vi "Next Buffer Size.vi"(3 "Min Size":i32=5, 4 "Times":u32[](array[numeric]), 5 "Buffer Duration (s)":dbl=2.0) -> (0 "Frequency (Hz)":dbl, 2 "Next buffer size":i32)   [LabVIEW 2009]
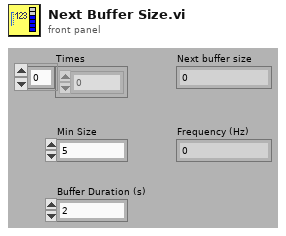
[diagram p1: front panel]
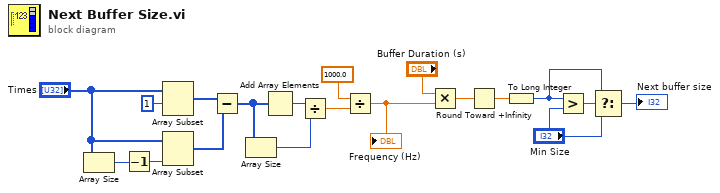
[diagram p0: block diagram]
diagram:
  n1 = Array Size(array="Times") -> (size(s)=w6:i32)
  n2 = Decrement(x=w6) -> (x-1=w5:i32)
  n3 = Array Subset(array="Times", index=1) -> (w10:u32[])  [unwired: 1 in]
  n4 = Array Subset(array="Times", length=w5) -> (w11:u32[])  [unwired: 1 in]
  n5 = Subtract(x=w10, y=w11) -> (x-y=w12:u32[])
  n6 = Array Size(array=w12) -> (size(s)=w14:i32)
  n7 = Add Array Elements(numeric array=w12) -> (sum=w13:u32)
  n8 = Divide(x=w13, y=w14) -> (x/y=w15:dbl)
  n9 = Divide(x=1000.0, y=w15) -> (x/y=w2:dbl)
  "Frequency (Hz)" <- w2
  n10 = Multiply(x="Buffer Duration (s)", y=w2) -> (x*y=w1:dbl)
  n11 = Round Toward +Infinity(x=w1) -> (ceil(x): smallest int >= x=w8:dbl)
  n12 = To Long Integer(number=w8) -> (32bit integer=w7:i32)
  n13 = Greater?(x=w7, y="Min Size") -> (0:w17:bool)
  n14 = Select(t=w7, s=w17, f="Min Size") -> (s? t:f=→"Next buffer size":i32)
